vi "Filter.vi"(8 "error in (no error)":errorcluster, 10 "Filter":u32(ring) items=["Off", "On"], 11 "VISA resource name":refnum<visa-resource-name>) -> (0 "error out":errorcluster, 3 "VISA resource name out":refnum<visa-resource-name>)   [LabVIEW 2017, in "Newport 1830-C.lvlib"]
doc: "1= use the slow filter to average to average the last 16 measurements\n2= us the medium filter to average the last 4 measurements\n3= no averaging is performed"
uses:
  Newport 1830-C.lvlib
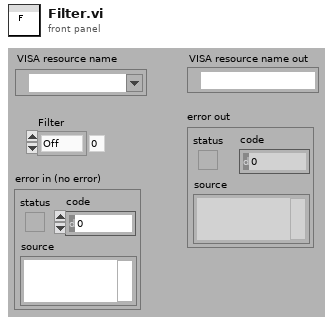
[diagram p1: front panel]
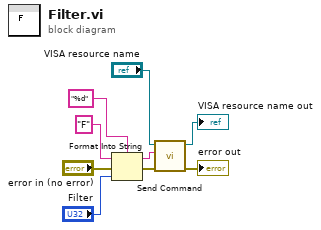
[diagram p0: block diagram]
diagram:
  n1 = Format Into String(format string="%d", initial string="F" ("command"), error in="error in (no error)", "Filter") -> (resulting string=w5:string, error out=w6:errorcluster)
  n2 = call "Send Command.vi"("error in (no error)"=w6, "write buffer"=w5, "VISA resource name In"="VISA resource name") -> ("error out"=→"error out":errorcluster, "VISA resource name out"=→"VISA resource name out":refnum<visa-resource-name>)  [unwired: 7 in]
